vi "TDMS Determine Sub-Folder.vi"(8 "error in (no error)":errorcluster, 10 "SN Limit":i32, 11 "MN Path":path) -> (0 "error out":errorcluster, 3 "TDMS Path":path)   [LabVIEW 2011]
uses:
  OpenG.LIB/array/array.llb/Remove Duplicates from 1D Array (String)__ogtk.vi
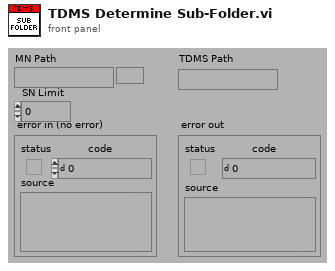
[diagram p1: front panel]
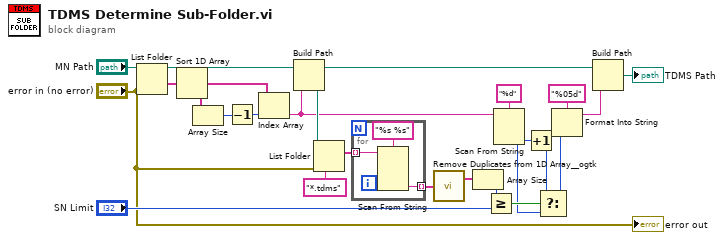
[diagram p0: block diagram]
diagram:
  n1 = List Folder(path="MN Path", error in="error in (no error)") -> (path out=w16:path, folder names=w23:string[])  [unwired: 2 in, 2 out]
  n2 = Sort 1D Array(array=w23) -> (sorted array=w22:string[])
  n3 = Array Size(array=w22) -> (size(s)=w21:i32)
  n4 = Decrement(x=w21) -> (x-1=w8:i32)
  n5 = Index Array(array=w22, index=w8) -> (element=w17:string)
  n6 = Build Path(base path=w16, name or relative path=w17) -> (appended path=w20:path)
  n7 = List Folder(path=w20, pattern="*.tdms", error in="error in (no error)") -> (filenames=w6:string[])  [unwired: 1 in, 3 out]
  n8 = for {
    tunnel: w6 -> [w26] mode=indexing
    tunnel: [w24] -> w5 mode=indexing
    n9 = Scan From String(format string="%s %s", input string=w26) -> (output 2=w24:string)  [unwired: 5 in, 3 out]
  }
  n10 = call-poly "Remove Duplicates from 1D Array__ogtk.vi"("Input Array"=w5) -> ("Output Array"=w4:string[])  [unwired: 1 out]
  n11 = Array Size(array=w4) -> (size(s)=w18:i32)
  n12 = Greater Or Equal?(x=w18, y="SN Limit") -> (x >= y?=w12:bool)
  n13 = Scan From String(format string="%d", input string=w17) -> (output 1=w11:i32)  [unwired: 3 in, 3 out]
  n14 = Increment(x=w11) -> (x+1=w10:i32)
  n15 = Select(t=w10, s=w12, f=w11) -> (s? t:f=w9:i32)
  n16 = Format Into String(format string="%05d", w9) -> (resulting string=w15:string)  [unwired: 2 in, 1 out]
  n17 = Build Path(base path=w16, name or relative path=w15) -> (appended path=→"TDMS Path":path)
  "error out" <- "error in (no error)"
